vi "Test basic.vi"() -> ()   [LabVIEW 2020]
uses:
  UI_Actor/UI_Actor Messages/UI_ShowIn_FreeWindow Msg/UI_ShowIn_FreeWindow Msg.lvclass
  UI_Actor/UI_Actor Messages/UI_Hide Msg/UI_Hide Msg.lvclass
  UI_Actor/UI_Actor Messages/UI_ShowIn_Subpanel Msg/UI_ShowIn_Subpanel Msg.lvclass
  UI_Actor/UI_Actor Messages/UI_Resize Msg/UI_Resize Msg.lvclass
  UI_Actor/UI_Actor/UI_Actor.lvclass
  UI_Actor/UI_Actor Messages/UI_KBB_Trig Msg/UI_KBB_Trig Msg.lvclass
  support/Actor Framework.lvlibp/1abvi3w/vi.lib/ActorFramework/Stop Msg/Stop Msg.lvclass
  UIA_ChildTest/UIA_ChildTest/UIA_ChildTest.lvclass
  support/Databox.lvlibp/TypesTools/Config/Config.lvclass
  UI_Actor/UI_Actor Messages/UI_AutoRefresh Msg/UI_AutoRefresh Msg.lvclass
  support/Databox.lvlibp/TypesTools/Data/Data.lvclass
  support/Databox.lvlibp/TypesTools/Data/TypeEnum.ctl
  D:/Projets/STEP AT/UI Actor/UI_Actor/UI_Actor/UI_Actor.lvclass
  UI_Actor/UI_Actor/ctl_AR_Mode.ctl
  UI_Actor/UI_Actor/ctl_AR_Parameters.ctl
panel:
  in  "Parameters":T1={"Write TipStrips with details (T)"=TRUE, "Write Captions with UserLabels (T)"=TRUE, "Mode (ind only)"=enum."Indicators only"}
  in  "KBB":bool
  in  "Actor Name":string
  in  "Remove from SP":bool
  in  "Units":string[](array[string])=["%", "km", "°C", "-", "", "", " ", "kV", "A"]
  in  "UserLab":string[](array[string])=["coucou 1", "coucou 2", "temp", "c chaud", "", "", " ", "yes!", "Clust num"]
  in  "SysLab":string[](array[string])=["ctl1", "ctl2", "indic1", "indic2", "ring", "enum", "slide", "Indic3 in tab ctl", "Clust num"]
  in  "Data":dbl[](array[numeric])=[15.6, 159.7, 27.8, 4.0, 0.0, 0.0, 20.0, 5.0, -3.0]
  in  "Resize":bool
  in  "ShowIn SP":bool
  in  "Hide":bool
  in  "Show free":bool
  in  "stop":bool
  # "AUTO REFRESH"
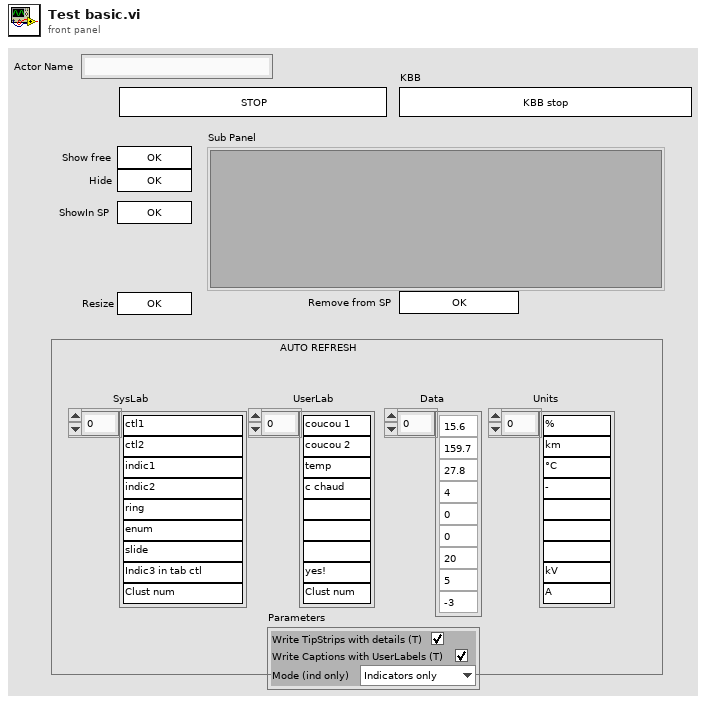
[diagram p1: front panel]
types:
  T1 = typedef "UI_Actor.lvlib/UI_Actor.lvclass/ctl_AR_Parameters.ctl" = cluster{"Write TipStrips with details (T)":bool, "Write Captions with UserLabels (T)":bool, "Mode (ind only)":T2}
  T2 = typedef "UI_Actor.lvlib/UI_Actor.lvclass/ctl_AR_Mode.ctl" = enum16{"Controls only", "Indicators only", "All"}
  T3 = cluster{"Ch.Conf":refnum<class "Config.lvclass">, "Data":refnum<class "Data.lvclass">[]}
  T4 = typedef "Databox.lvlibp/Data.lvclass/TypeEnum.ctl" = enum16{"Boolean", "SByte", "Byte", "Int16", "UInt16", "Int32", "UInt32", "Int64", "UInt64", "Float", "Double", "String", "DateTime", "ByteString", "Array of Boolean", "Array of SByte", "Array of Byte", "Array of Int16", "Array of UInt16", "Array of Int32", "Array of UInt32", "Array of Int64", "Array of UInt64", "Array of Float", "Array of Double", "Array of String", "Array of DateTime", "Array of ByteString", "Matrix of Boolean", "Matrix of SByte", "Matrix of Byte", "Matrix of Int16", "Matrix of UInt16", "Matrix of Int32", "Matrix of UInt32", "Matrix of Int64", "Matrix of UInt64", "Matrix of Float", "Matrix of Double", "Matrix of String ", "Matrix of DateTime", "Matrix of ByteString"}
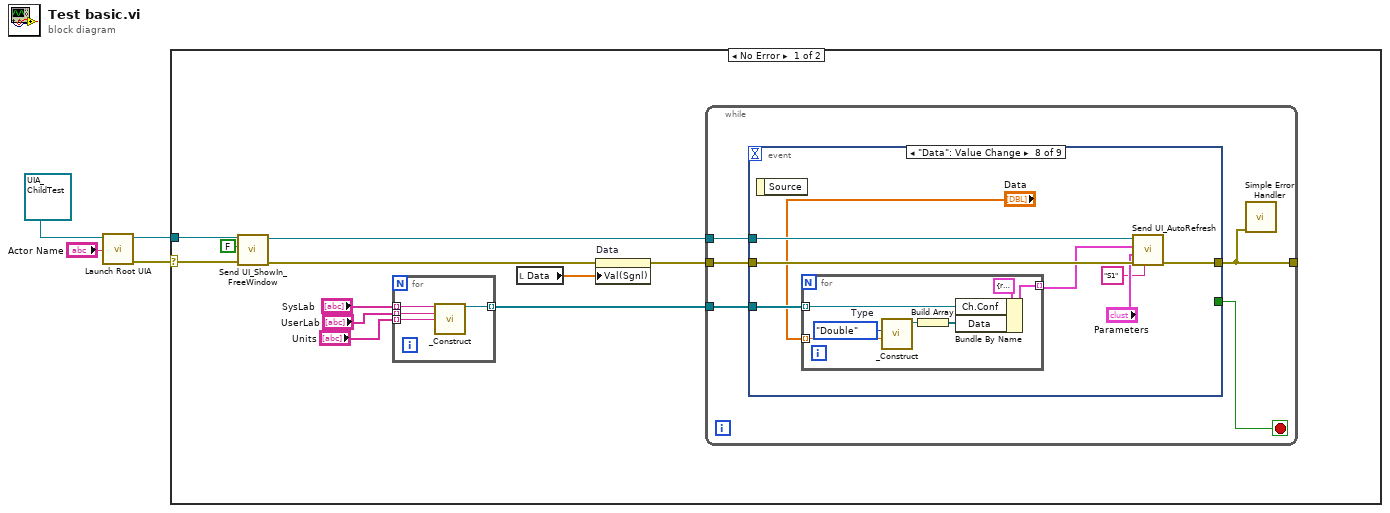
[diagram p0: block diagram]
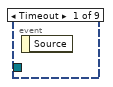
[diagram p2: hidden frame]
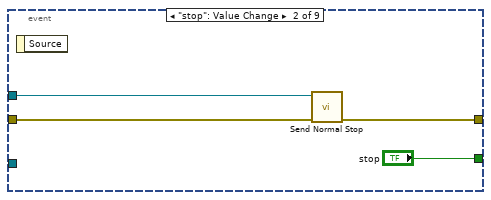
[diagram p3: hidden frame]
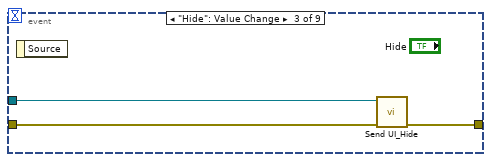
[diagram p4: hidden frame]
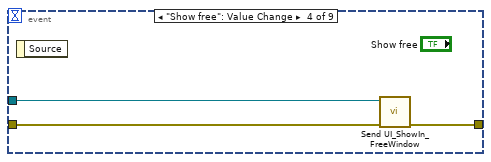
[diagram p5: hidden frame]
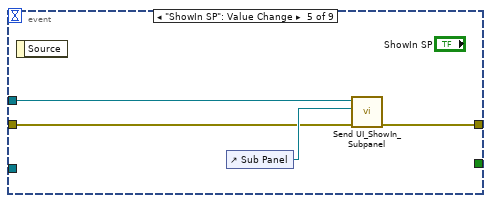
[diagram p6: hidden frame]
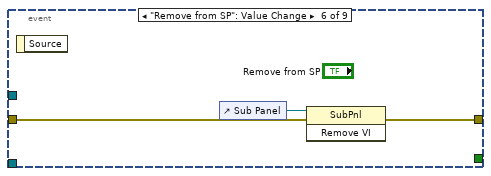
[diagram p7: hidden frame]
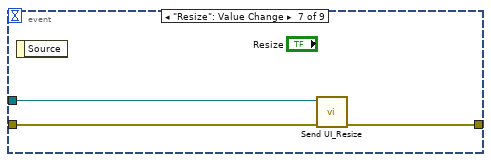
[diagram p8: hidden frame]
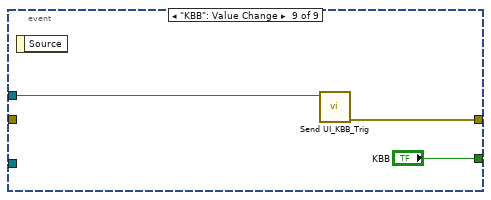
[diagram p9: hidden frame]
diagram:
  n1 = call "Launch Root UIA.vi"("Actor Name"="Actor Name", "UI_Actor in"=refnum<class "UIA_ChildTest.lvclass"> refnum ("UIA_ChildTest.lvlib:UIA_ChildTest.lvclass")) -> ("error out"=w3:errorcluster, "Actor's Enqueuer"=w4:refnum<class "Message Enqueuer.lvclass">)  [unwired: 8 in]
  n2 = case shown="No Error" w3 {
    selector: w3 -> [w15 _]
    tunnel: w4 -> [w9 _]
    frame No Error {
      n3 = call "Send UI_ShowIn_FreeWindow.vi"("error in (no error)"=w15, "Standard/Max (T=Max)"=FALSE, "Message Enqueuer"=w9) -> ("error out"=w7:errorcluster, "Message Enqueuer out"=w14:refnum<class "Message Enqueuer.lvclass">)  [unwired: 7 in]
      n4 = for {
        tunnel: [w19] -> w5 mode=indexing
        tunnel: "SysLab" -> [w18] mode=indexing
        tunnel: "UserLab" -> [w17] mode=indexing
        tunnel: "Units" -> [w16] mode=indexing
        n5 = call "_Construct.vi"("System Label"=w18, "User Label"=w17, "Unit"=w16) -> ("Ch.Conf out"=w19:refnum<class "Config.lvclass">)  [unwired: 11 in, 1 out]
      }
      n6 = local read "Data"() -> (w8:dbl[])
      n7 = property on="Data" class="Arr (strict)"(error in=w7, "Val(Sgnl)"=w8) -> (error out=w6:errorcluster)  [unwired: 1 in, 1 out]
      n8 = while {
        tunnel: w14 -> [w23]
        tunnel: [w21] -> _
        tunnel: w6 -> [w22]
        tunnel: w5 -> [w20]
        stop <- w24 stop-if-true
        n9 = event shown="[7] \"Data\": Value Change" {
          selector: _ -> [_ _ _ _ _ _ _ _ _]
          dyn-events: _ -> [_ _ _ _ _ _ _ _ _]
          timeout: _ -> [_ _ _ _ _ _ _ _ _]
          tunnel: [_ "stop" _ _ _ _ _ _ "KBB"] -> w24
          tunnel: w23 -> [_ w25 w31 w34 w38 _ w44 w52 w61]
          tunnel: [_ w26 w29 w32 w35 w39 w42 w50 w60] -> w21
          tunnel: w22 -> [_ w27 w30 w33 w36 w40 w43 w51 _]
          tunnel: w20 -> [_ _ _ _ _ _ _ w47 _]
          event Timeout {
            n10 = event-data() -> ()  [unwired: 1 in, 1 out]
          }
          event "stop": Value Change {
            n11 = event-data() -> ()  [unwired: 1 in, 1 out]
            n12 = call "Send Normal Stop.vi"("error in (no error)"=w27, "Message Enqueuer"=w25) -> ("error out"=w26:errorcluster)  [unwired: 9 in]
          }
          event "Hide": Value Change {
            n13 = event-data() -> ()  [unwired: 1 in, 1 out]
            n14 = call "Send UI_Hide.vi"("error in (no error)"=w30, "Message Enqueuer"=w31) -> ("error out"=w29:errorcluster)  [unwired: 8 in, 1 out]
          }
          event "Show free": Value Change {
            n15 = event-data() -> ()  [unwired: 1 in, 1 out]
            n16 = call "Send UI_ShowIn_FreeWindow.vi"("error in (no error)"=w33, "Message Enqueuer"=w34) -> ("error out"=w32:errorcluster)  [unwired: 8 in, 1 out]
          }
          event "ShowIn SP": Value Change {
            n17 = event-data() -> ()  [unwired: 1 in, 1 out]
            n18 = control-ref of="Sub Panel"() -> (w37:refnum<vi>)
            n19 = call "Send UI_ShowIn_Subpanel.vi"("error in (no error)"=w36, "Sub Panel"=w37, "Message Enqueuer"=w38) -> ("error out"=w35:errorcluster)  [unwired: 7 in, 1 out]
          }
          event "Remove from SP": Value Change {
            n20 = event-data() -> ()  [unwired: 1 in, 1 out]
            n21 = control-ref of="Sub Panel"() -> (w41:refnum<vi>)
            n22 = invoke class="SubPnl" method="Remove VI"(reference=w41, error in=w40) -> (error out=w39:errorcluster)  [unwired: 1 in, 2 out]
          }
          event "Resize": Value Change {
            n23 = event-data() -> ()  [unwired: 1 in, 1 out]
            n24 = call "Send UI_Resize.vi"("error in (no error)"=w43, "Message Enqueuer"=w44) -> ("error out"=w42:errorcluster)  [unwired: 8 in, 1 out]
          }
          event "Data": Value Change {
            n25 = event-data() -> ()  [unwired: 1 in, 1 out]
            n26 = for {
              tunnel: [w58] -> w48 mode=indexing
              tunnel: w47 -> [w57] mode=indexing
              tunnel: "Data" -> [w53] mode=indexing
              w54 = TypeEnum."Double"  # Type
              n27 = call "_Construct.vi"("Value"=w53, "Type"=w54) -> ("Ch.TData out"=w56:refnum<class "Data.lvclass">)  [unwired: 8 in, 1 out]
              n28 = Build Array(w56) -> (w55:refnum<class "Data.lvclass">[])
              n29 = Bundle By Name(cluster=T3 {"Ch.Conf"=refnum, "Data"=[]} ("Cluster"), "Ch.Conf"=w57, "Data"=w55) -> (w58:T3)
            }
            n30 = call "Send UI_AutoRefresh.vi"("Sourcer name"="S1", "error in (no error)"=w51, "Parameters (Tipstrips,Captions,All)"="Parameters", "Data chunk"=w48, "Message Enqueuer"=w52) -> ("error out"=w50:errorcluster)  [unwired: 5 in, 1 out]
          }
          event "KBB": Value Change {
            n31 = event-data() -> ()  [unwired: 1 in, 1 out]
            n32 = call "Send UI_KBB_Trig.vi"("Message Enqueuer"=w61) -> ("error out"=w60:errorcluster)  [unwired: 9 in, 1 out]
          }
        }
        n33 = call <vilib>:"Simple Error Handler.vi"("error in (no error)"=w21) -> ()  [unwired: 4 in, 5 out]
      }
    }
    frame Error {
    }
  }
